vi "XIPIN_High_Speed_SelectIO_Wizard_2_0.vi"   [LabVIEW 2017]
doc: "The High Speed SelectIO Wizard creates a HDL file (Verilog ) that contains IO and clocking logic such as RX/TX_BITSLICE, BITSLICE_CONTROL and PLL blocks customized to the user's interface requirements. Pin LOC update in this wizard updates the RTL to provide required connectivity among blocks\n------------------------------------\n<b>Need License</b> : No"
uses:
  <vilib>/rvi/XilinxIP/XIPIN_XNode/niFpgaXIPIN.xnode
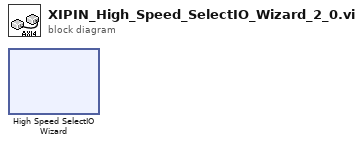
[diagram p0: block diagram]
diagram:
  n1 = xnode ("High Speed SelectIO Wizard")() -> ()
